vi "Insight_Peak_Finder.vi"(5 "threshold":dbl=0.5 format="%0.2f", 6 "width":i32=3 min=3, 7 "peaks/valleys":enum32{"Peaks", "Valleys"}(ring)=enum."Valleys", 8 "error in (no error)":errorcluster, 9 "input data":dbl[](array[numeric]), 10 "Stop Value":i32=1, 11 "Start Value":i32) -> (0 "error out":errorcluster, 2 "Locations":dbl[](array[numeric]))   [LabVIEW 2011]
uses:
  <vilib>/Analysis/NI_AAL_SigProc.lvlib
panel:
  out "Raw Input":dbl[](graph)
  out "Amplitudes":dbl[](array[numeric])
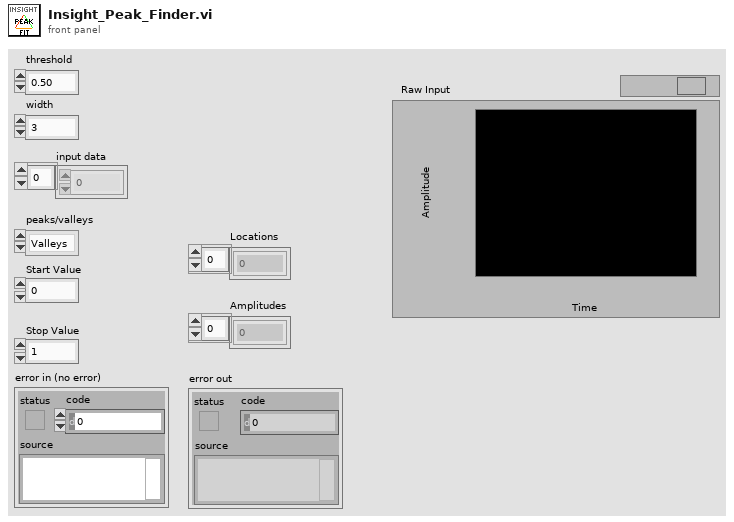
[diagram p1: front panel]
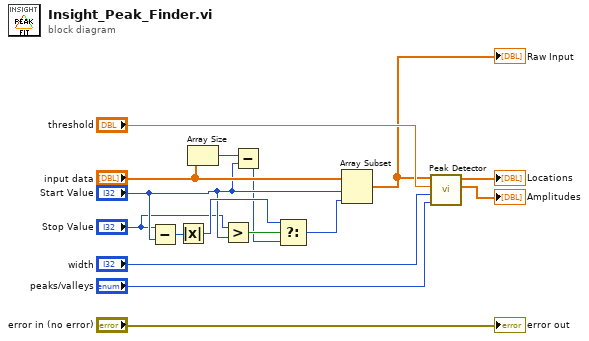
[diagram p0: block diagram]
diagram:
  n1 = Subtract(x="Stop Value", y="Start Value") -> (x-y=w13:i32)
  n2 = Absolute Value(x=w13) -> (abs(x)=w9:i32)
  n3 = Array Size(array="input data") -> (size(s)=w6:i32)
  n4 = Greater?(x="Stop Value", y="Start Value") -> (0:w10:bool)
  n5 = Subtract(x=w6, y="Start Value") -> (x-y=w4:i32)
  n6 = Select(t=w9, s=w10, f=w4) -> (s? t:f=w8:i32)
  n7 = Array Subset(array="input data", index="Start Value", length=w8) -> (w2:dbl[])
  "Raw Input" <- w2
  n8 = call <vilib>:"Peak Detector.vi"("peaks/valleys"="peaks/valleys", "width"="width", "threshold"="threshold", "X"=w2) -> ("Amplitudes"=→"Amplitudes":dbl[], "Locations"=→"Locations":dbl[])  [unwired: 3 in, 3 out]
  "error out" <- "error in (no error)"
